vi "DistanceStatus.vi"(1 "Status i":bool[](array[boolean]), 2 "Y":i32[](array[numeric]), 3 "X":i32[](array[numeric])) -> (0 "Status i+1":bool[](array[boolean]))   [LabVIEW 2014]
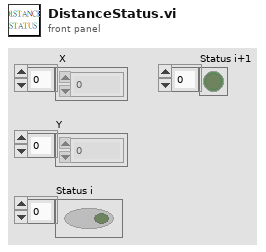
[diagram p1: front panel]
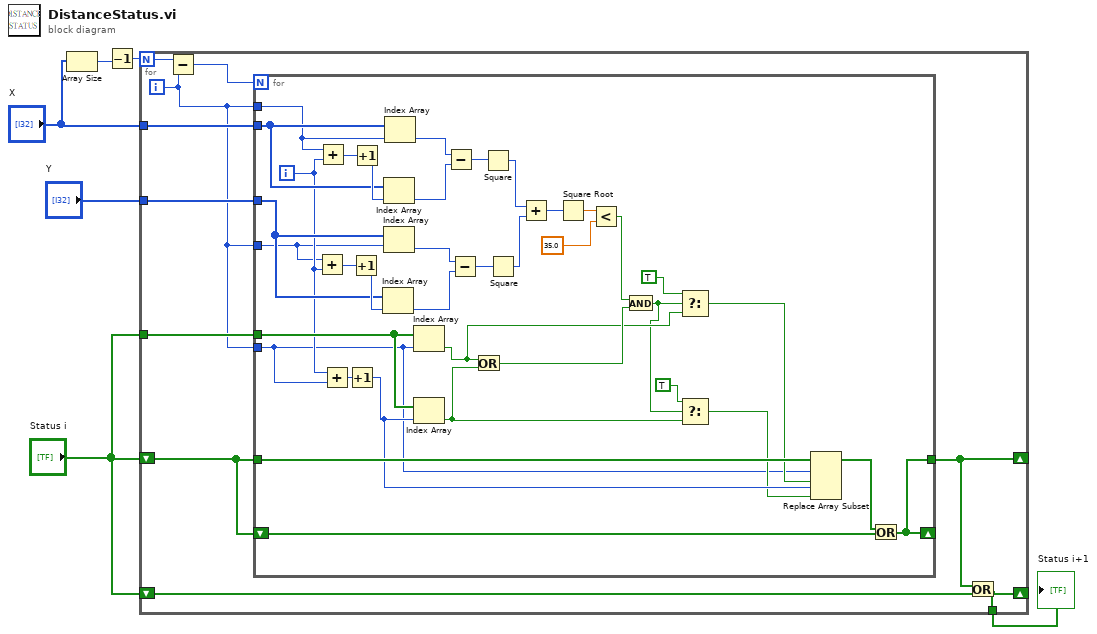
[diagram p0: block diagram]
diagram:
  n1 = Array Size(array="X") -> (size(s)=w1:i32)
  n2 = Decrement(x=w1) -> (x-1=w2:i32)
  n3 = for {
    N: w2 -> [w16]
    tunnel: "X" -> [w15]
    tunnel: "Y" -> [w14]
    tunnel: "Status i" -> [w13]
    shift-right: [w12] -> _
    shift-left: "Status i" -> [w8]
    shift-right: [w9] -> _
    shift-left: "Status i" -> [w11]
    tunnel: [w9] -> w6
    i -> [w7]
    n4 = Subtract(x=w16, y=w7) -> (x-y=w10:i32)
    n5 = for {
      N: w10 -> [_]
      tunnel: w7 -> [w19]
      tunnel: w15 -> [w51]
      tunnel: w14 -> [w48]
      tunnel: w7 -> [w17]
      tunnel: w13 -> [w31]
      tunnel: w8 -> [w28]
      tunnel: [w21] -> w12
      shift-right: [w21] -> _
      shift-left: w8 -> [w22]
      tunnel: w7 -> [w18]
      i -> [w20]
      n6 = Add(x=w18, y=w20) -> (x+y=w49:i32)
      n7 = Add(x=w19, y=w20) -> (x+y=w53:i32)
      n8 = Add(x=w20, y=w17) -> (x+y=w37:i32)
      n9 = Increment(x=w37) -> (x+1=w26:i32)
      n10 = Increment(x=w49) -> (x+1=w50:i32)
      n11 = Increment(x=w53) -> (x+1=w52:i32)
      n12 = Index Array(array=w48, index=w50) -> (element=w46:i32)
      n13 = Index Array(array=w51, index=w52) -> (element=w44:i32)
      n14 = Index Array(array=w48, index=w18) -> (element=w47:i32)
      n15 = Index Array(array=w51, index=w19) -> (element=w45:i32)
      n16 = Index Array(array=w31, index=w17) -> (element=w30:bool)
      n17 = Index Array(array=w31, index=w26) -> (element=w29:bool)
      n18 = Subtract(x=w45, y=w44) -> (x-y=w43:i32)
      n19 = Subtract(x=w47, y=w46) -> (x-y=w42:i32)
      n20 = Or(x=w30, y=w29) -> (x .or. y?=w36:bool)
      n21 = Square(x=w43) -> (x^2=w41:i32)
      n22 = Square(x=w42) -> (x^2=w40:i32)
      n23 = Add(x=w41, y=w40) -> (x+y=w39:i32)
      n24 = Square Root(x=w39) -> (sqrt(x)=w32:dbl)
      n25 = Less?(x=w32, y=35.0) -> (x < y?=w35:bool)
      n26 = And(x=w35, y=w36) -> (x .and. y?=w24:bool)
      n27 = Select(t=TRUE, s=w24, f=w30) -> (s? t:f=w27:bool)
      n28 = Select(t=TRUE, s=w24, f=w29) -> (s? t:f=w25:bool)
      n29 = Replace Array Subset(array=w28, new element #1=w27, index #1=w17, new element #2=w25, index #2=w26) -> (w23:bool[])
      n30 = Or(x=w23, y=w22) -> (x .or. y?=w21:bool[])
    }
    n31 = Or(x=w12, y=w11) -> (x .or. y?=w9:bool[])
  }
  "Status i+1" <- w6
